vi "Keyboard Shortcuts.vi"(7 "QRD":T2, 8 "error in":errorcluster, 11 "VKey":T1) -> (0 "error out":errorcluster, 3 "Discard?":bool, 5 "QRD Out":T2)   [LabVIEW 2025]
uses:
  Builds/Queue Wrappers.lvlibp
  Builds/Queue Wrappers.lvlibp/Q Packet.ctl
  Controls/Queues-Refs-Data.ctl
  <vilib>/event_ctls.llb/eventvkey.ctl
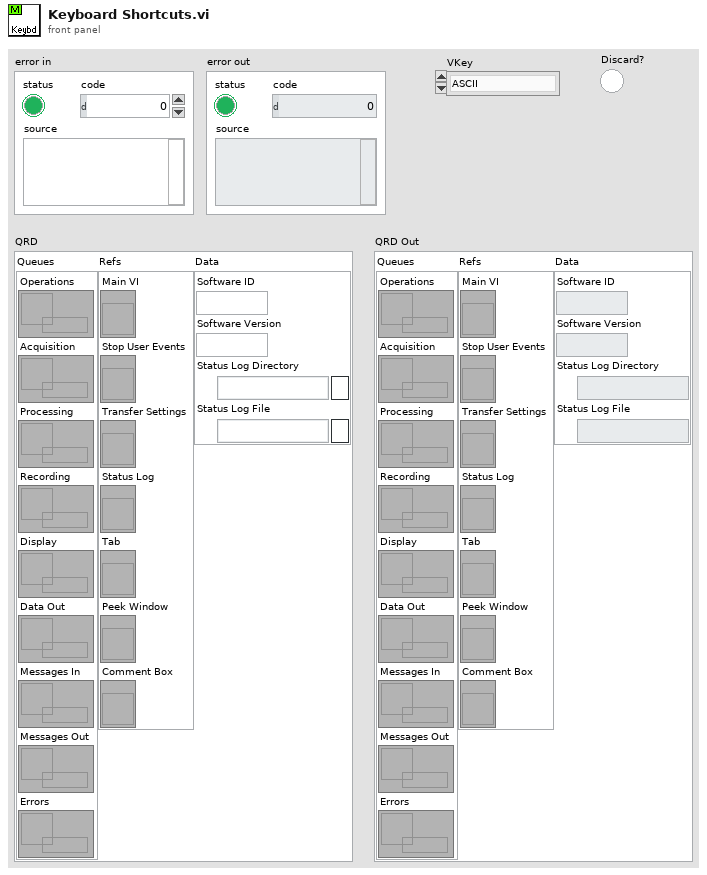
[diagram p1: front panel]
types:
  T1 = typedef "eventvkey.ctl" = enum16{"ASCII", "Enter", "Return", "Shift", "Ctrl", "Alt", "Cmd", "Opt", "Caps", "NumLock", "Clear", "Break", "Up", "Down", "Left", "Right", "Insert", "Delete", "Home", "End", "PageUp", "PageDown", "Escape", "Help", "Pause", "ScrollLock", "F1", "F2", "F3", "F4", "F5", "F6", "F7", "F8", "F9", "F10", "F11", "F12", "F13", "F14", "F15", "F16", "F17", "F18", "F19", "F20", "F21", "F22", "F23", "F24", "Play", "VolumeUp", "VolumeDown", "Mute", "Two Byte Char"}
  T2 = typedef "Queues-Refs-Data.ctl" = cluster{"Queues":cluster{"Operations":refnum<queue>, "Acquisition":refnum<queue>, "Processing":refnum<queue>, "Recording":refnum<queue>, "Display":refnum<queue>, "Data Out":refnum<queue>, "Messages In":refnum<queue>, "Messages Out":refnum<queue>, "Errors":refnum<queue>}, "Refs":cluster{"Main VI":refnum<vi>, "Stop User Events":refnum<vi>, "Transfer Settings":refnum<vi>, "Status Log":refnum<vi>, "Tab":refnum<vi>, "Peek Window":refnum<vi>, "Comment Box":refnum<vi>}, "Data":cluster{"Software ID":string, "Software Version":string, "Status Log Directory":path, "Status Log File":path}}
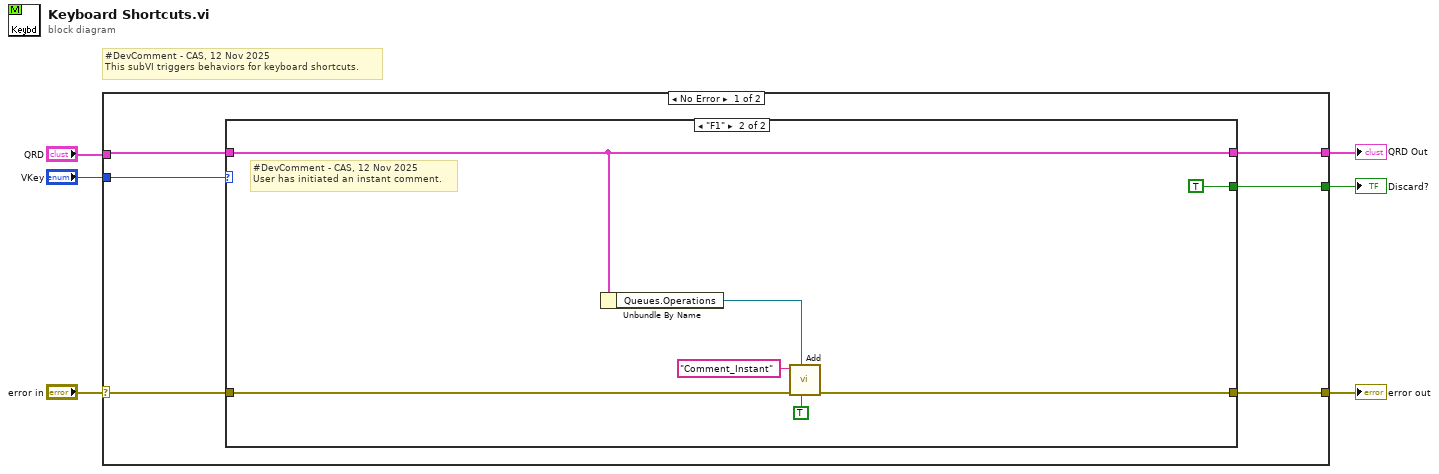
[diagram p0: block diagram]
diagram:
  # "#DevComment - CAS, 12 Nov 2025\nThis subVI triggers behaviors for keyboard shortcuts."
  n1 = case shown="No Error" "error in" {
    selector: "error in" -> [w10 w22]
    tunnel: [w12 w23] -> w6
    tunnel: "QRD" -> [w11 w23]
    tunnel: [w9 w22] -> w3
    tunnel: "VKey" -> [w8 _]
    tunnel: [w7 _] -> w1
    frame No Error {
      n2 = case shown="\"F1\"" w8 {
        tunnel: [w14 w19] -> w12
        tunnel: w11 -> [w14 w19]
        tunnel: w10 -> [w13 w21]
        tunnel: [w13 w20] -> w9
        tunnel: [_ TRUE] -> w7
        frame Default {
        }
        frame "F1" {
          # "#DevComment - CAS, 12 Nov 2025\nUser has initiated an instant comment."
          n3 = Unbundle By Name(w19) -> ("Queues.Operations"=w18:refnum<queue>)
          n4 = call "Add.vi"("Priority Message"=TRUE, "Q Ref In"=w18, "error in"=w21, "Packet ID"="Comment_Instant") -> ("error out"=w20:errorcluster)  [unwired: 4 in, 3 out]
        }
      }
    }
    frame Error {
    }
  }
  "error out" <- w3
  "QRD Out" <- w6
  "Discard?" <- w1
